vi "ASI Get Num Of Connected Cameras.vi"() -> (0 "error out":errorcluster, 3 "function return":i32)   [LabVIEW 2023, in "ASICamera2_no_err.lvlib"]
doc: "ASICAMERA_API int ASIGetNumOfConnectedCameras();"
uses:
  ASICamera2_no_err.lvlib
  ASICamera2.dll
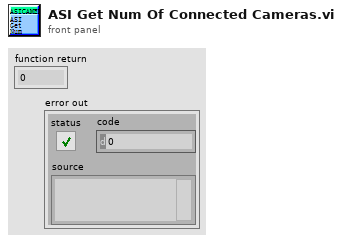
[diagram p1: front panel]
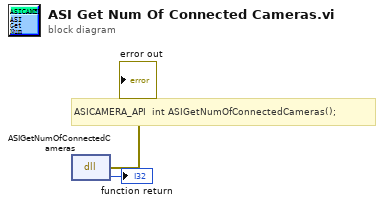
[diagram p0: block diagram]
diagram:
  # "ASICAMERA_API  int ASIGetNumOfConnectedCameras();"
  n1 = dll-call lib="W:/Quant_Opt_Group/Group/Alex/LabviewDAQ-master/ConcreteClasses/ConcreteInstrumentClasses/CameraClasses/ZWO_ASI_LV/Labview_ASI_demo_64bit_221128/user.lib/ASICamera2_no_err/ASICamera2.*" fn="ASIGetNumOfConnectedCameras"() -> (error out=→"error out":errorcluster, →"function return":i32)  [unwired: 3 in, 1 out]
